vi "Pass State Machine.vi"   [LabVIEW 2013]
uses:
  typedefs/fg_typedef.ctl
  typedefs/subStates.ctl
  UberCode Suffield Philification/typedefs/DevRef Type.ctl
panel:
  # "A State Machine to Handle Passing"
types:
  T1 = typedef "subStates.ctl" = enum16{"null", "wait", "driver control", "auto", "manual override", "hold position", "rotate", "pickup", "pass", "load", "goto shoot", "shoot high goal", "shoot low goal", "cancel arm", "cancel shooter", "end"}
  T2 = typedef "fg_typedef.ctl" = enum16{"Get", "Set"}
  T3 = typedef "DevRef Type.ctl" = enum16{"Shooter Solenoid", "Latch Solenoid", "Right Up Sensor", "Right Down Sensor", "Hold Sensor", "Arm Encoder"}
  T4 = typedef "WPI_DigitalInputDevRef.ctl" = cluster{"DevStatus":errorcluster, "DIO Channel":T5, "Digital Module":T6}
  T5 = typedef "FPGA_DIOChannel.ctl" = enum8{"DIO 1", "DIO 2", "DIO 3", "DIO 4", "DIO 5", "DIO 6", "DIO 7", "DIO 8", "DIO 9", "DIO 10", "DIO 11", "DIO 12", "DIO 13", "DIO 14", "Invalid"}
  T6 = typedef "FPGA_TypedefDigitalModule.ctl" = enum16{"Digital Module 1", "Digital Module 2"}
  T7 = typedef "WPI_EncoderDevRef.ctl" = cluster{"DevStatus":errorcluster, "EncoderIndex":T8, "CounterIndex":T9, "DistancePerCount":dbl, "Decoding Type":T10}
  T8 = typedef "FPGA_EncoderIdx.ctl" = enum8{"Enc 0", "Enc 1", "Enc 2", "Enc 3", "Invalid"}
  T9 = typedef "FPGA_CounterCtrSystemIndex.ctl" = enum8{"Ctr 0", "Ctr 1", "Ctr 2", "Ctr 3", "Ctr 4", "Ctr 5", "Ctr 6", "Ctr 7", "Invalid"}
  T10 = typedef "WPI_EncoderType.ctl" = enum16{"1x", "2x", "4x"}
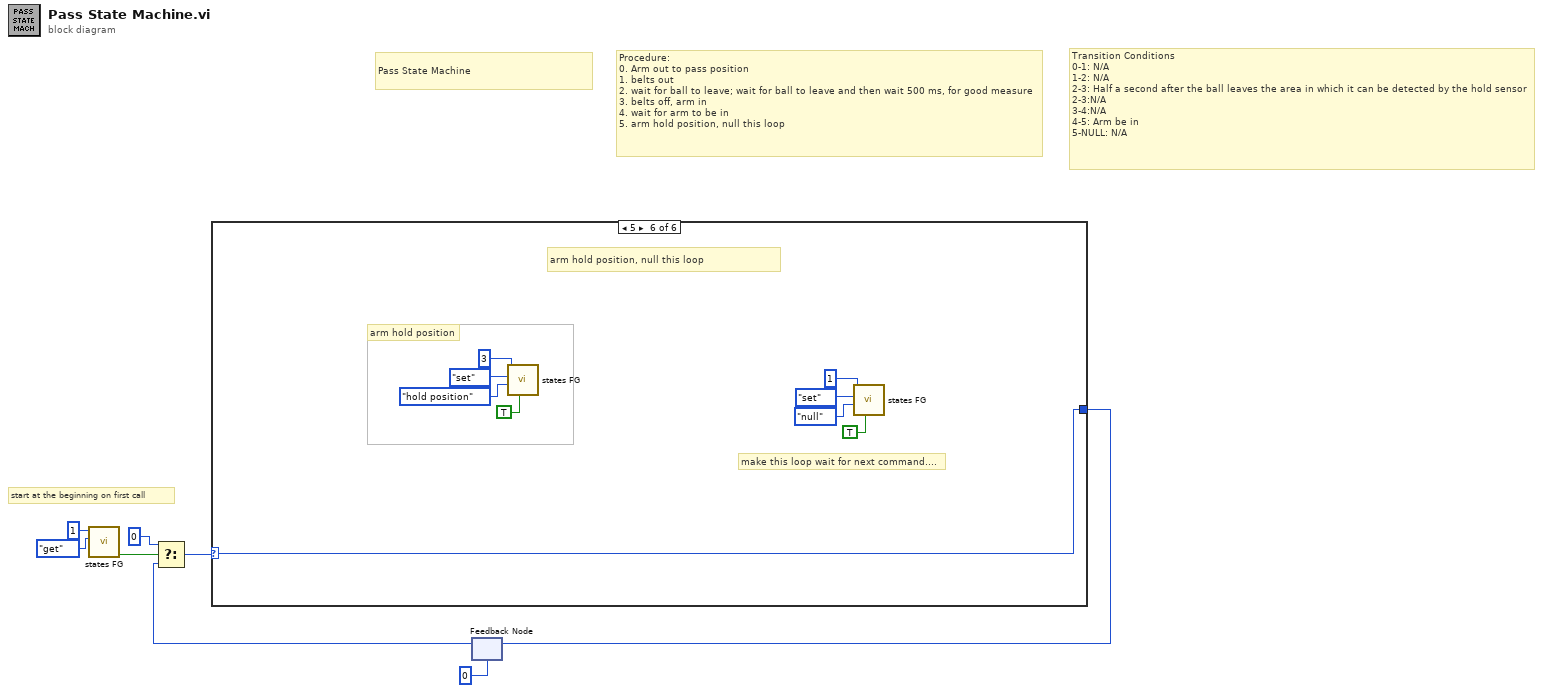
[diagram p0: block diagram]
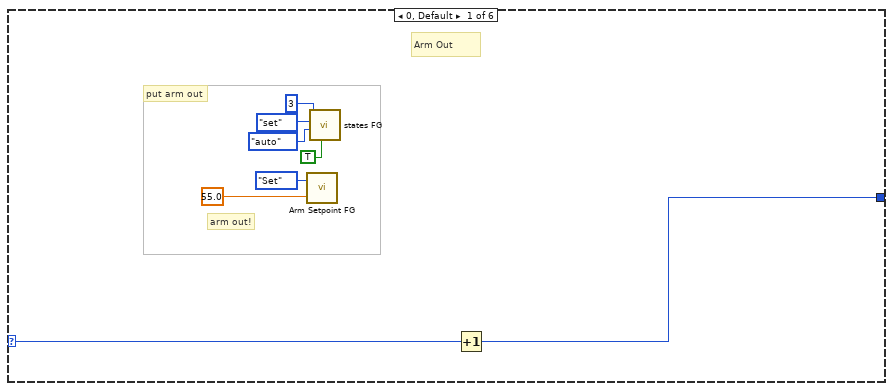
[diagram p2: hidden frame]
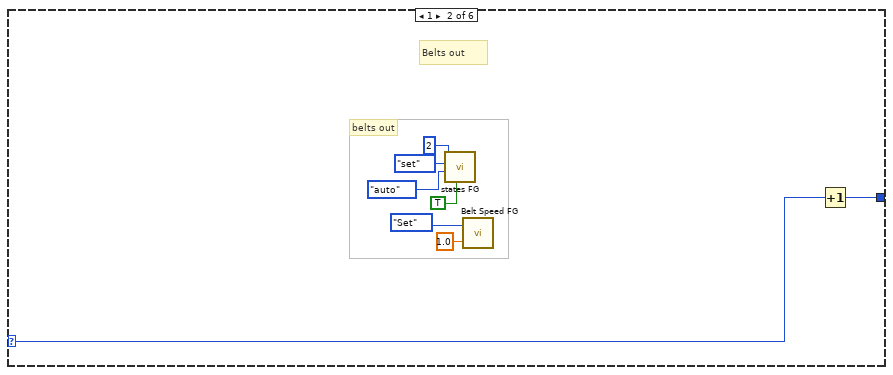
[diagram p3: hidden frame]
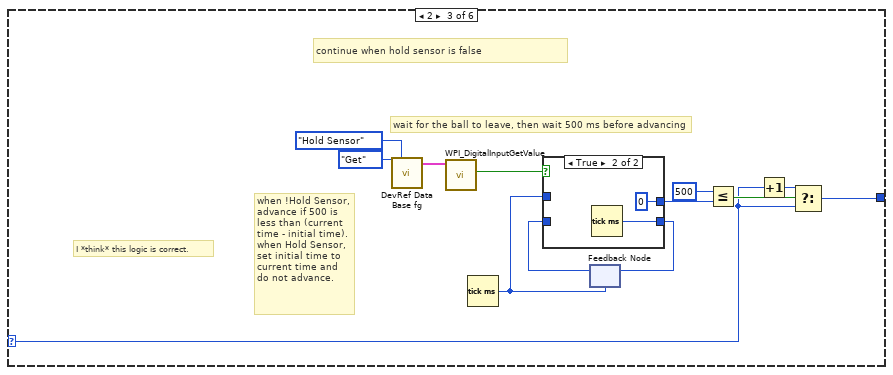
[diagram p4: hidden frame]
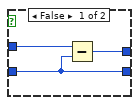
[diagram p5: hidden frame]
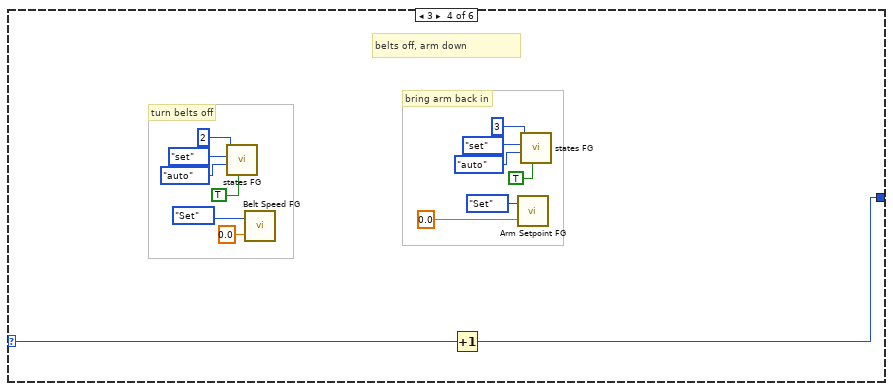
[diagram p6: hidden frame]
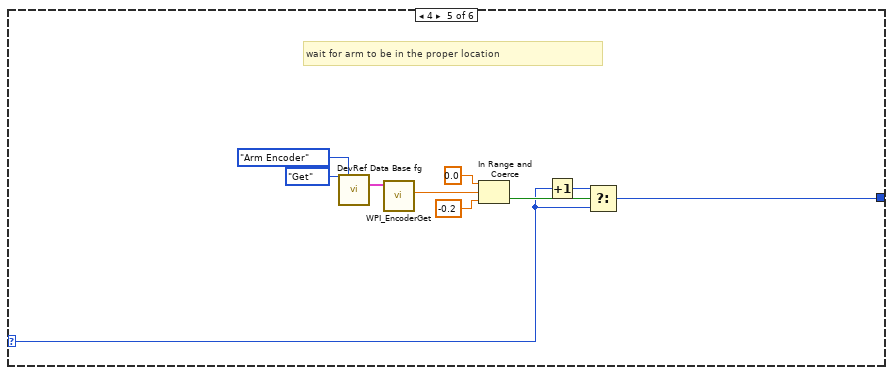
[diagram p7: hidden frame]
diagram:
  # "Transition Conditions\n0-1: N/A\n1-2: N/A\n2-3: Half a second after the ball leaves the area in which it can be detected by the hold sensor\n2-3:N/A\n3-4:N/A\n4-5: Arm be in\n5-NULL: N/A"
  # "Procedure:\n0. Arm out to pass position\n1. belts out\n2. wait for ball to leave; wait for ball to leave and then wait 500 ms, for good measure\n3. belts off, arm in\n4. wait for arm to be in\n5. arm hold position, null this loop"
  # "Pass State Machine"
  # "start at the beginning on first call"
  n1 = call "states FG.vi"("menu (get)"=enum16{"set", "get"}."get", "Loop ID"=1) -> ("first call?"=w1:bool)  [unwired: 6 in, 3 out]
  n2 = feedback #1(u8 0) -> (w4:u8)
  n3 = Select(t=u8 0, s=w1, f=w4) -> (s? t:f=w3:u8)
  n4 = case shown="5" w3 {
    selector: w3 -> [w11 w18 w26 w46 w59 w67]
    tunnel: [w10 w17 w25 w45 w57 w67] -> w7
    frame 0, Default {
      # "put arm out"
      # "Arm Out"
      # "arm out!"
      n5 = call "Arm Setpoint FG.vi"("Setpoint In"=55.0, "Menu"=fg_typedef."Set") -> ()  [unwired: 1 out]
      n6 = call "states FG.vi"("exit in"=TRUE, "subState in"=subStates."auto", "menu (get)"=enum16{"set", "get"}."set", "Loop ID"=3) -> ()  [unwired: 4 in, 4 out]
      n7 = Increment(x=w11) -> (x+1=w10:u8)
    }
    frame 1 {
      # "belts out"
      # "Belts out"
      n8 = call "states FG.vi"("exit in"=TRUE, "subState in"=subStates."auto", "menu (get)"=enum16{"set", "get"}."set", "Loop ID"=2) -> ()  [unwired: 4 in, 4 out]
      n9 = call "Belt Speed FG.vi"("Speed In"=1.0, "Menu"=fg_typedef."Set") -> ()  [unwired: 1 out]
      n10 = Increment(x=w18) -> (x+1=w17:u8)
    }
    frame 2 {
      # "continue when hold sensor is false"
      # "I *think* this logic is correct."
      # "when !Hold Sensor,\nadvance if 500 is\nless than (current\ntime - initial time).\nwhen Hold Sensor,\nset initial time to\ncurrent time and\ndo not advance."
      # "wait for the ball to leave, then wait 500 ms before advancing"
      n11 = call "DevRef Data Base fg.vi"("Menu"=fg_typedef."Get", "DevRef to Get"=DevRef_Type."Hold Sensor") -> ("Selected Sensor"=w28:T4)  [unwired: 23 in, 2 out]
      n12 = call <vilib>:"WPI_DigitalInputGetValue.vi"("DigitalInputDevRef"=w28) -> ("Value"=w30:bool)  [unwired: 8 in, 2 out]
      n13 = Tick Count (ms)() -> (millisecond timer value=w34:u32)
      n14 = feedback #2(w34) -> (w33:u32)
      n15 = case shown="True" w30 {
        tunnel: [w40 w42] -> w37
        tunnel: w33 -> [w40 _]
        tunnel: [w39 u32 0] -> w36
        tunnel: w34 -> [w38 _]
        frame False {
          n16 = Subtract(x=w38, y=w40) -> (x-y=w39:u32)
        }
        frame True {
          n17 = Tick Count (ms)() -> (millisecond timer value=w42:u32)
        }
      }
      n18 = feedback-in #2(w37) -> ()
      n19 = Less Or Equal?(x=u32 500, y=w36) -> (x <= y?=w32:bool)
      n20 = Increment(x=w26) -> (x+1=w31:u8)
      n21 = Select(t=w31, s=w32, f=w26) -> (s? t:f=w25:u8)
    }
    frame 3 {
      # "turn belts off"
      # "bring arm back in"
      # "belts off, arm down"
      n22 = call "states FG.vi"("exit in"=TRUE, "subState in"=subStates."auto", "menu (get)"=enum16{"set", "get"}."set", "Loop ID"=2) -> ()  [unwired: 4 in, 4 out]
      n23 = call "Belt Speed FG.vi"("Speed In"=0.0, "Menu"=fg_typedef."Set") -> ()  [unwired: 1 out]
      n24 = Increment(x=w46) -> (x+1=w45:u8)
      n25 = call "Arm Setpoint FG.vi"("Setpoint In"=0.0, "Menu"=fg_typedef."Set") -> ()  [unwired: 1 out]
      n26 = call "states FG.vi"("exit in"=TRUE, "subState in"=subStates."auto", "menu (get)"=enum16{"set", "get"}."set", "Loop ID"=3) -> ()  [unwired: 4 in, 4 out]
    }
    frame 4 {
      # "wait for arm to be in the proper location"
      n27 = call "DevRef Data Base fg.vi"("Menu"=fg_typedef."Get", "DevRef to Get"=DevRef_Type."Arm Encoder") -> ("Selected Encoder"=w64:T7)  [unwired: 23 in, 2 out]
      n28 = call <vilib>:"WPI_EncoderGet.vi"("EncoderDevRef"=w64) -> ("Distance"=w63:dbl)  [unwired: 5 in, 5 out]
      n29 = In Range and Coerce(upper limit=0.0, x=w63, lower limit=-0.2) -> (In Range?=w60:bool)  [unwired: 1 out]
      n30 = Increment(x=w59) -> (x+1=w58:u8)
      n31 = Select(t=w58, s=w60, f=w59) -> (s? t:f=w57:u8)
    }
    frame 5 {
      # "arm hold position"
      # "make this loop wait for next command...."
      # "arm hold position, null this loop"
      n32 = call "states FG.vi"("exit in"=TRUE, "subState in"=subStates."hold position", "menu (get)"=enum16{"set", "get"}."set", "Loop ID"=3) -> ()  [unwired: 4 in, 4 out]
      n33 = call "states FG.vi"("exit in"=TRUE, "subState in"=subStates."null", "menu (get)"=enum16{"set", "get"}."set", "Loop ID"=1) -> ()  [unwired: 4 in, 4 out]
    }
  }
  n34 = feedback-in #1(w7) -> ()
